vi "Peek Open.vi"(11 "adstar in":refnum<class "NI_Robotics_AnytimeDStar.lvclass">) -> (2 "node ref out":refnum<data-value>, 3 "adstar out":refnum<class "NI_Robotics_AnytimeDStar.lvclass">)   [LabVIEW 2017, in "NI_Robotics_AnytimeDStar.lvclass"]
uses:
  <vilib>/robotics/Navigation/Anytime D Star/NI_Robotics_AnytimeDStar.lvclass
  <vilib>/robotics/Navigation/shared/MapNode/AbstractDstarNode/NI_Robotics_AbstractDstarNode.lvclass
  <vilib>/robotics/Navigation/Anytime D Star/NI_Robotics_AnytimeDStar.lvclass/NI_Robotics_AnytimeDStar.ctl
  <vilib>/robotics/Navigation/shared/MapNode/AbstractMapNode/NI_Robotics_AbstractMapNode.lvclass
  <vilib>/robotics/Navigation/shared/Priority Queue/NI_Robotics_Priority Queue.lvclass
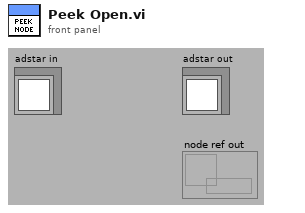
[diagram p1: front panel]
types:
  T1 = typedef "NI_Robotics_Priority Queue.lvclass/Open List Element.ctl" = cluster{"f":dbl, "g":dbl, "node Ref":refnum<data-value>}
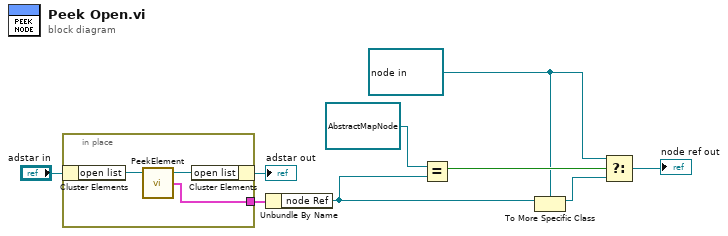
[diagram p0: block diagram]
diagram:
  w2 = refnum<data-value> refnum ("node ref out")
  n1 = in-place {
    in-place-border: [w10] -> w7
    n2 = in-place-cluster #1("adstar in") -> ("open list"=w12:refnum<class "NI_Robotics_Priority Queue.lvclass">)
    n3 = call <vilib>:"PeekElement.vi"("Astar Open List in"=w12) -> ("Open List Element"=w10:T1, "Astar Open List out"=w11:refnum<class "NI_Robotics_Priority Queue.lvclass">)  [unwired: 2 in, 1 out]
    n4 = in-place-cluster #1("open list"=w11) -> (→"adstar out":refnum<class "NI_Robotics_AnytimeDStar.lvclass">)
  }
  n5 = Unbundle By Name(w7) -> ("node Ref"=w6:refnum<data-value>)
  n6 = Equal?(x=refnum<data-value> refnum ("node Ref"), y=w6) -> (x = y?=w3:bool)
  n7 = To More Specific Class(target class=w2, reference=w6) -> (specific class reference=w5:refnum<data-value>)  [unwired: 1 in, 1 out]
  n8 = Select(t=w2, s=w3, f=w5) -> (s? t:f=→"node ref out":refnum<data-value>)
